vi "Editor Folder.vi"(10 "Value Type String":string, 11 "Value Name":string) -> (2 "Type Only Folder":string, 3 "Name & Type Folder":string)   [LabVIEW 2020, in "FlexBlocks.lvlib"]
uses:
  FlexBlocks.lvlib
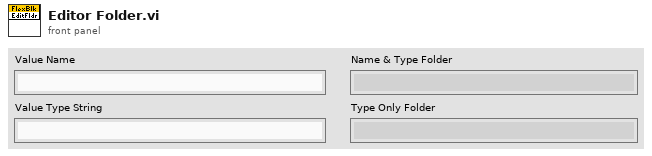
[diagram p1: front panel]
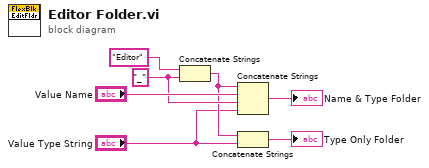
[diagram p0: block diagram]
diagram:
  w5 = "_" ("string")
  n1 = Concatenate Strings("Editor" ("string"), w5) -> (w3:string)
  n2 = Concatenate Strings(w3, "Value Name", w5, "Value Type String") -> (→"Name & Type Folder":string)
  n3 = Concatenate Strings(w3, "Value Type String") -> (→"Type Only Folder":string)
